vi "FPGAFilter.vi"(7 "filter on":bool, 10 "coeff addr":i16, 11 "x":fxp<+/-,24,4>) -> (3 "y":fxp<+/-,24,4> format="%.22g")   [LabVIEW 2019]
doc: "FIR Direct Form filter\n\n# Channels: 1\n\nInput word length: 16\nOutput data format (wl.iwl): Q16.2\nGain is processed on the host."
uses:
  <vilib>/Platform/TimedLoop/XDataNode/timing_clust.ctl
  <vilib>/Platform/TimedLoop/XDataNode/nitl_modes.ctl
  <vilib>/Platform/TimedLoop/XDataNode/wakeup.ctl
  <vilib>/rvi/FXPMathLib/FxpConvert/subVIs/nifxpmath_Convert_SimConfig.ctl
  <vilib>/fxp/LVFixedPointQuantizationPolicyTypeDef.ctl
  <vilib>/fxp/LVFixedPointOverflowPolicyTypeDef.ctl
  <vilib>/rvi/DataTransferAndStorage/Container/Common/niFpgaContainerGetUniqueNameForEmu.vi
  <vilib>/rvi/DataTransferAndStorage/Container/Common/niFpgaContainerSetEmuInfo.vi
  <vilib>/rvi/eio/common/nirviEmuReportErrorAndStop.vi
  <vilib>/rvi/Emulation/niFpgaSctlEmulationGetInTimedLoop.vi
  <vilib>/rvi/Emulation/niFpgaEmulationReportErrorSimple.vi
  <vilib>/rvi/Emulation/niFpgaGetClockAttributes.vi
  <vilib>/rvi/Emulation/niFpgaCriticalErrorInLSC.vi
  <vilib>/rvi/Memory/Memory_Emulation/nirvimemoryEmulation.vi
  <vilib>/rvi/Memory/Memory_Emulation/nirvimemoryFastEmulation.vi
  <vilib>/rvi/Memory/Memory_Emulation/niFpgaMemoryEmulationCacheClearOnFirstRun.vi
  <vilib>/rvi/Memory/Memory_Emulation/nirvimemoryEmulationManagerCache_MakeExclusive.vi
  <vilib>/rvi/Memory/Memory_Emulation/niFpgaMemoryEmulationValidateCache.vi
  <vilib>/rvi/Memory/Memory_Emulation/nirvimemoryEmulationManagerCache_InsertValue.vi
  <vilib>/Utility/error.llb/Clear Errors.vi
  <vilib>/rvi/Memory/Memory_Emulation/nirvimemoryEmulationManagerCache_ReleaseExclusive.vi
  <vilib>/rvi/Memory/Memory_Emulation/nirvimemoryEmulationManagerCache_GetValue.vi
  <vilib>/rvi/Emulation/niFpgaEmulationIsFPGAContextNoSignature.vi
  <vilib>/rvi/Memory/Memory_Emulation/nirvimemoryEmulationManagerCache_SetValue.vi
  <vilib>/rvi/Emulation/niFpgaSctlEmulationResourceMgr.vi
  <vilib>/rvi/interface/RandomDataEmulation/niFpgaRandomDataHandleErrors.vi
  <vilib>/rvi/FXPMathLib/FxpConvert/simVIs/DllFxpConvertTemp_sub.vi
  <vilib>/rvi/LocalResourceManager/LocalResourceManager.xnode
  <vilib>/Platform/TimedLoop/XDataNode/XDataNode.xnode
  <vilib>/rvi/DataTransferAndStorage/Container/XNode/niFpgaContainer.xnode
  <vilib>/rvi/FXPMathLib/FxpAdd/XNode/nifxpmath_Add.xnode
  <vilib>/rvi/interface/RandomDataEmulation/nirviRandomDataFpgaReadWriteTemplate.vi
  <vilib>/rvi/FXPMathLib/FxpMul/XNode/nifxpmath_Multiplier.xnode
  <vilib>/rvi/FXPMathLib/FxpConvert/XNode/nifxpmath_Convert.xnode
  <vilib>/Platform/TimedLoop/XDataNode/XDNodeRunTimeDep.lvlib
  <vilib>/rvi/FXPMathLib/sim/FxpSim.dll
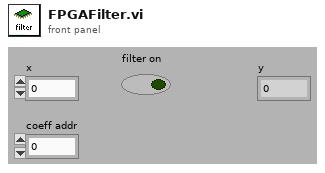
[diagram p1: front panel]
types:
  T1 = typedef "XDNodeRunTimeDep.lvlib/timing_clust.ctl" = cluster{"Expected End [f-1]":u64, "Actual End [f-1]":u64, "Finished Late? [f-1]":bool, "Expected End [i-1]":u64, "Actual End [i-1]":u64, "Finished Late? [i-1]":bool, "Expected Start [i]":u64, "Actual Start [i]":u64, "Expected Start [f]":u64, "Actual Start [f]":u64, "Source Name":string, "Structure Name":string, "Period":i64, "Deadline":i64, "Offset":i64, "Start":i64, "Priority":i32, "Timeout":i32, "Mode":T2, "Wakeup Reason":T3, "Error":errorcluster, "Source Type":string, "Secondary Source Type":string, "Global End Time":u64, "Global Start Time":u64, "Frame Duration":u64, "Iteration Duration":u64, "Assigned CPU":i32, "I/O Scan Engine Mode":u32}
  T2 = typedef "XDNodeRunTimeDep.lvlib/nitl_modes.ctl" = enum32{"No Change", "Process missed periods, maintain original phase", "Discard missed periods, maintain original phase", "Process missed periods, ignore original phase", "Discard missed periods, ignore original phase"}
  T3 = typedef "XDNodeRunTimeDep.lvlib/wakeup.ctl" = enum32{"Normal", "Aborted", "Asynchronous wakeup", "Timing source error", "Timed loop error", "Timeout"}
  T4 = cluster{"RDEn?":bool, "coefAddr":u16, "WREn?":bool, "memAddr":u16, "stop":bool}
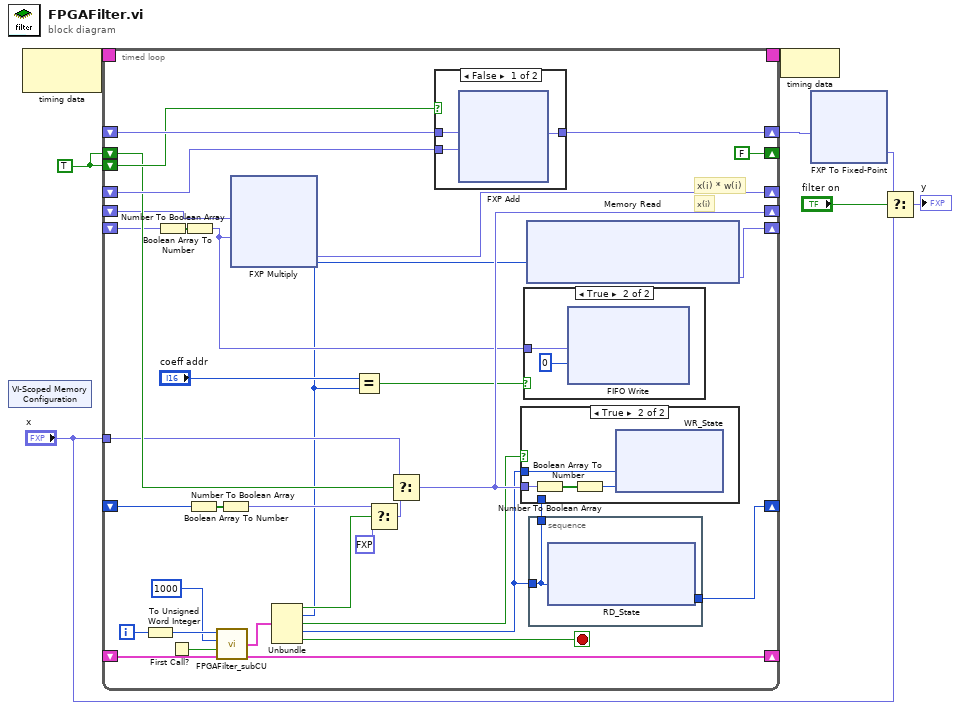
[diagram p0: block diagram]
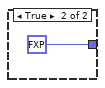
[diagram p4: hidden frame]
diagram:
  w8 = TRUE
  n1 = xnode "VI-Scoped Memory Configuration"() -> ()  [unwired: 1 out]
  n2 = node-c288() -> (w2:T1)  [unwired: 1 in]
  n3 = timed-loop "Main Loop" {
    shift-right: [w18] -> _
    shift-left: _ -> [w17]
    shift-right: [w13] -> _
    shift-left: _ -> [w14]
    shift-right: [w43] -> _
    shift-left: _ -> [w24]
    shift-right: [w27] -> w7
    shift-left: _ -> [w41]
    shift-right: [w23] -> _
    shift-left: _ -> [w42]
    shift-right: [w39] -> _
    shift-left: _ -> [w38]
    shift-right: [FALSE] -> _
    shift-left: w8 -> [w30]
    shift-left: w8 -> [w32]
    tunnel: "x" -> [w21]
    timing: w2 -> [_]
    timing-out: [_] -> w1
    i -> [w25]
    stop <- w35 stop-if-true
    # "x(i) * w(i)"
    # "x(i)"
    n4 = To Unsigned Word Integer(number=w25) -> (unsigned 16bit integer=w40:u16)
    n5 = Number To Boolean Array(number=w14) -> (Boolean array=w15:bool[])
    n6 = First Call?() -> (First Call?: T/F=w37:bool)
    n7 = Boolean Array To Number(Boolean array=w15) -> (number=w12:fxp<+/-,24,4>)
    n8 = Number To Boolean Array(number=w17) -> (Boolean array=w19:bool[])
    n9 = call "FPGAFilter_subCU.vi"("states"=w38, "global reset"=w37, "filter length"=1000, "index"=w40) -> ("states"=w39:cluster{"addr start":u16, "first run?":bool}, "control info"=w29:T4)  [unwired: 6 out]
    n10 = Boolean Array To Number(Boolean array=w19) -> (number=w16:fxp<+/-,24,4>)
    n11 = xnode "FXP Multiply"("x"=w24, "y"=w12) -> ("x*y"=w23:fxp<+/-,32,4>)
    n12 = Unbundle(w29) -> ("RDEn?"=w20:bool, "coefAddr"=w10:u16, "WREn?"=w36:bool, "memAddr"=w28:u16, "stop"=w35:bool)
    n13 = Equal?(x="coeff addr", y=w10) -> (x = y?=w9:bool)
    n14 = Select(t=w16, s=w20, f=fxp<+/-,24,4> 0.0 ("InZero")) -> (s? t:f=w33:fxp<+/-,24,4>)
    n15 = Select(t=w21, s=w30, f=w33) -> (s? t:f=w43:fxp<+/-,24,4>)
    n16 = case shown="False" w32 {
      tunnel: [w52 fxp<+/-,32,4> 0.0] -> w27
      tunnel: w42 -> [w54 _]
      tunnel: w41 -> [w53 _]
      frame False {
        n17 = xnode "FXP Add"("x"=w53, "y"=w54) -> ("x+y"=w52:fxp<+/-,32,4>)
      }
      frame True {
      }
    }
    n18 = case shown="True" w9 {
      tunnel: w12 -> [_ w44]
      frame False {
      }
      frame True {
        n19 = xnode ("FIFO Write")("Element"=w44, "Timeout"=0) -> ()  [unwired: 1 in, 2 out]
      }
    }
    n20 = xnode ("Memory Read")("Address"=w10) -> ("Data"=w13:fxp<+/-,24,4>)  [unwired: 1 in, 1 out]
    n21 = stacked-sequence "MemRDCase" {
      tunnel: [w47] -> w18
      tunnel: w28 -> [w46]
      tunnel: [w46] -> w26
      frame #0 {
        n22 = xnode ("RD_State")("Address"=w46) -> ("Data"=w47:u32)  [unwired: 1 in, 1 out]
      }
    }
    n23 = case "MemWRCase" shown="True" w36 {
      tunnel: w43 -> [_ w49]
      tunnel: w28 -> [_ w51]
      tunnel: w26 -> [_ _]
      frame False {
      }
      frame True {
        n24 = Number To Boolean Array(number=w49) -> (Boolean array=w50:bool[])
        n25 = Boolean Array To Number(Boolean array=w50) -> (number=w48:u32)
        n26 = xnode ("WR_State")("Address"=w51, "Data"=w48) -> ()  [unwired: 1 in, 1 out]
      }
    }
  }
  n27 = node-c288(w1) -> ()
  n28 = xnode "FXP To Fixed-Point"("x"=w7) -> ("y"=w5:fxp<+/-,24,4>)
  n29 = Select(t=w5, s="filter on", f="x") -> (s? t:f=→"y":fxp<+/-,24,4>)
